vi "Initialize.vi"(8 "error in":errorcluster) -> (0 "error out":errorcluster)   [LabVIEW 2020, in "Hardware.lvlib"]
uses:
  Hardware.lvlib
  Messaging/Message FGV Actions.ctl
panel:
  # "HW Handler: Initialize"
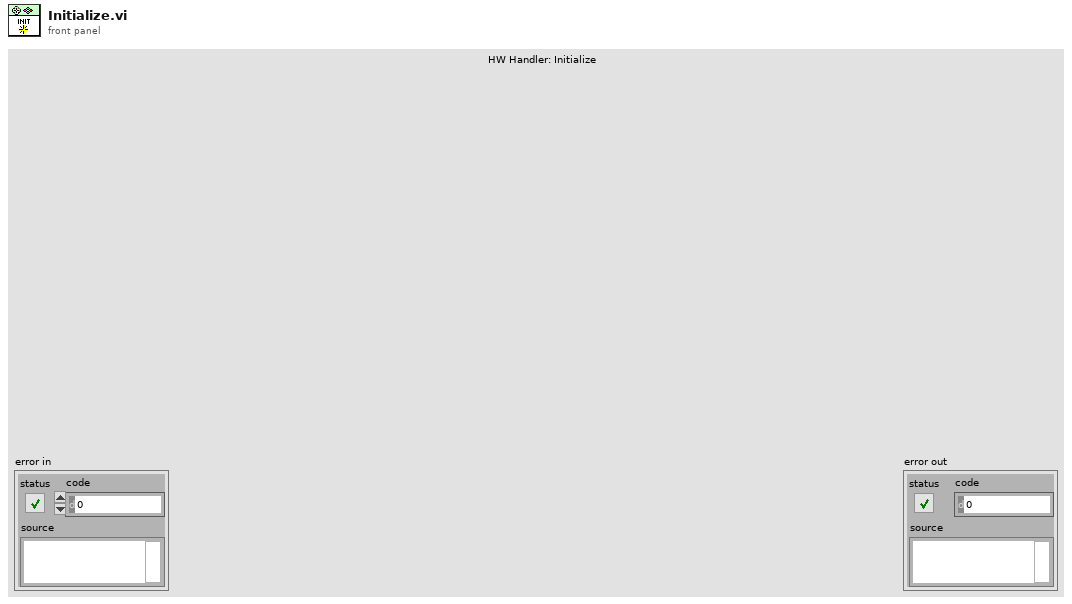
[diagram p1: front panel]
types:
  T1 = typedef "Hardware.lvlib/Message FGV Actions.ctl" = enum16{"Get", "Obtain", "Release", "Flush"}
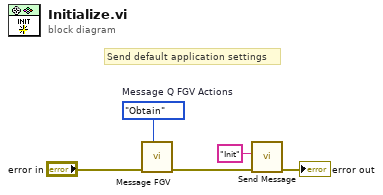
[diagram p0: block diagram]
diagram:
  w5 = Message_FGV_Actions."Obtain"  # Message Q FGV Actions
  # "Send default application settings"
  n1 = call "Message FGV.vi"("Message Q FGV Actions"=w5, "error in"="error in") -> ("error out"=w3:errorcluster)  [unwired: 6 in, 3 out]
  n2 = call "Send Message.vi"("error in"=w3, "Command"="Init") -> ("error out"=→"error out":errorcluster)  [unwired: 9 in]
